vi "Deqeue UI Element.vi"(8 "error in":errorcluster) -> (0 "error out":errorcluster, 1 "Data":variant, 2 "Message":string)   [LabVIEW 2024, in "User Interface Control.lvlib"]
uses:
  User Interface Control.lvlib
  Tester Internal Communication/Queues - Get.vi
  Tester Internal Communication/Tester InterComm.lvlib
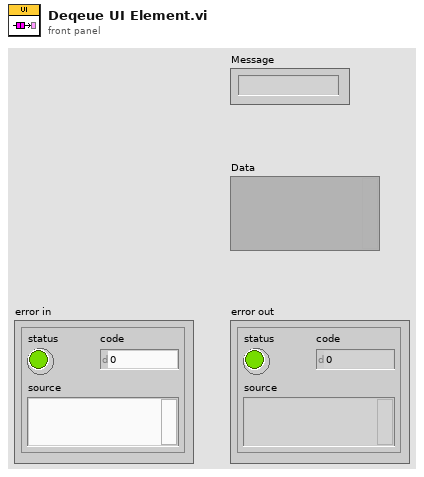
[diagram p1: front panel]
types:
  T1 = typedef "Tester InterComm.lvlib/Process Queues.ctl" = cluster{"UI":refnum<queue>, "Tester Requests":refnum<queue>}
  T2 = typedef "Tester InterComm.lvlib/QMH Item.ctl" = cluster{"Message":string, "Data":variant}
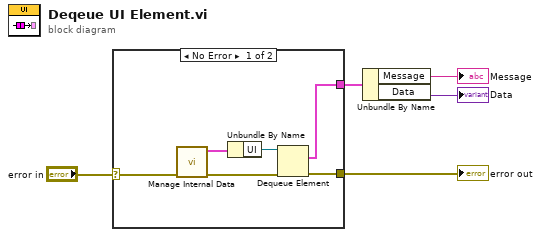
[diagram p0: block diagram]
diagram:
  n1 = case shown="No Error" "error in" {
    selector: "error in" -> [w8 w12]
    tunnel: [w7 w12] -> w4
    tunnel: [w6 _] -> w3
    frame No Error {
      n2 = call-poly "Manage Internal Data.vi"("error in"=w8) -> ("error out"=w9:errorcluster, "Queues Out"=w11:T1)  [unwired: 9 in]
      n3 = Unbundle By Name(w11) -> ("UI"=w10:refnum<queue>)
      n4 = Dequeue Element(queue=w10, error in (no error)=w9) -> (element=w6:T2, error out=w7:errorcluster)  [unwired: 1 in, 2 out]
    }
    frame Error {
    }
  }
  "error out" <- w4
  n5 = Unbundle By Name(w3) -> ("Message"=→"Message":string, "Data"=→"Data":variant)
